vi "FileSave.vi"(8 "error in (no error)":errorcluster, 10 "Process":refnum<vi>, 11 "Parameters In":refnum<vi>) -> (0 "error out":errorcluster)   [LabVIEW 2016]
uses:
  controls/process.ctl
  <vilib>/silver_ctls/ArrayMatrixCluster/Real Matrix NI_Silver.ctl
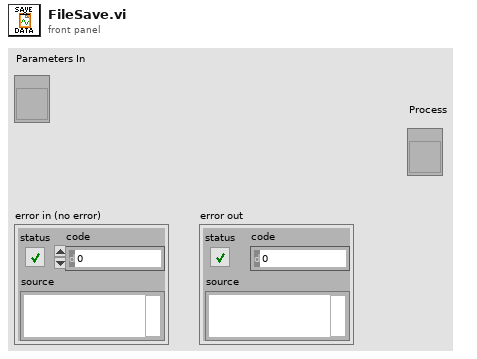
[diagram p1: front panel]
types:
  T1 = typedef "process.ctl" = cluster{"Sample":u16, "Lambda":u16, "Stabilizing":u16, "Status":u8, "Estimated Time":dbl, "Samples":T2, "Data":T2, "Lambda-Index":dbl, "Graph":bool}
  T2 = typedef "Real Matrix NI_Silver.ctl" = dbl[][]
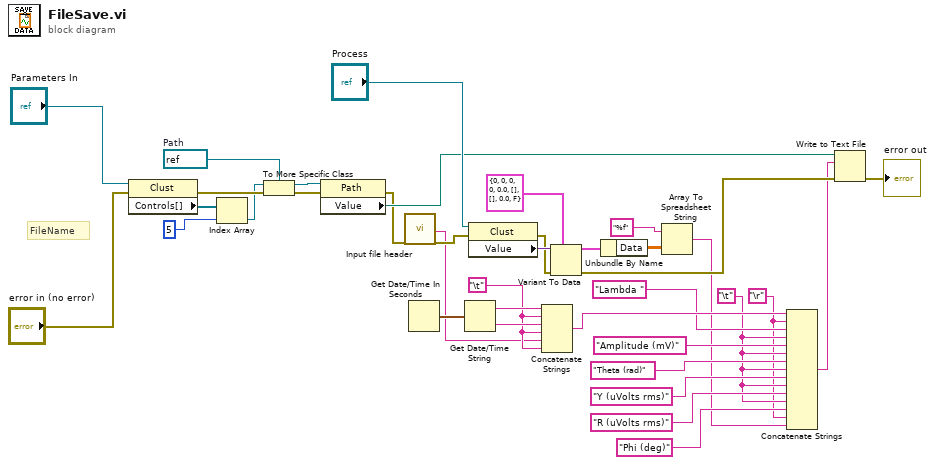
[diagram p0: block diagram]
diagram:
  w7 = "\t"
  w5 = "\r"
  w24 = "\t"
  w36 = refnum<vi> refnum  # Path
  # "FileName"
  n1 = property class="Clust"(reference="Parameters In", error in="error in (no error)") -> (error out=w33:errorcluster, "Controls[]"=w29:refnum<vi>[])  [unwired: 1 out]
  n2 = Index Array(array=w29, index=5) -> (element=w32:refnum<vi>)
  n3 = To More Specific Class(target class=w36, reference=w32, error in=w33) -> (specific class reference=w34:refnum<vi>, error out=w37:errorcluster)
  n4 = property class="Path"(reference=w34, error in=w37) -> (error out=w2:errorcluster, "Value"=w3:path)  [unwired: 1 out]
  n5 = call "Input file header"("error in (no error)"=w2) -> ("Header"=w1:string, "error out"=w17:errorcluster)  [unwired: 1 in, 16 out]
  n6 = Get Date/Time In Seconds() -> (seconds since 1Jan1904=w27:timestamp)
  n7 = Get Date/Time String(seconds (now)=w27) -> (date string=w26:string, time string=w25:string)  [unwired: 2 out]
  n8 = property class="Clust"(reference="Process", error in=w17) -> (error out=w20:errorcluster, "Value"=w21:variant)  [unwired: 1 out]
  n9 = Concatenate Strings(w26, w24, w25, w24, w1, w24) -> (w13:string)
  n10 = Variant To Data(error in=w20, type=T1 {"Sample"=0, "Lambda"=0, "Stabilizing"=0, "Status"=0, "Estimated Time"=0.0, "Samples"=[], "Data"=[], "Lambda-Index"=0.0, "Graph"=FALSE} ("Process"), Variant=w21) -> (data=w18:T1, error out=w16:errorcluster)
  n11 = Unbundle By Name(w18) -> ("Data"=w15:T2)
  n12 = Array To Spreadsheet String(array=w15, 3:"%f") -> (spreadsheet string=w4:string)  [unwired: 1 in]
  n13 = Concatenate Strings(w13, w5, "Lambda ", w7, "Amplitude (mV)", w7, "Theta (rad)", w7, "Y (uVolts rms)", w7, "R (uVolts rms)", w7, "Phi (deg)", w5, w4) -> (w14:string)
  n14 = Write to Text File(file (use dialog)=w3, text=w14, error in=w16) -> (error out=→"error out":errorcluster)  [unwired: 1 in, 2 out]
